vi "自定义成像色谱20200214.vi"(3 "错误输入（无错误）":errorcluster) -> (6 "Color palette":T1(array[cluster]), 7 "生成的色谱条":T2(plugin-control))   [LabVIEW 2018]
uses:
  <vilib>/vision/NI_Vision_Development_Module.lvlib
panel:
  out "对应幅值":dbl[](array[numeric])=[0.0, 0.0, 0.0, 0.0, 255.0, 128.0, 255.0] format="%#.1f%%"
  in  "确 定":bool
  in  "色阶":u32=6 min=2 max=32
  in  "自定义颜色梯度":u32[](array[colorbox])=[8388608, 16744448, 14276864, 32768, 8454143, 16512, 16777215]
  # "自定义显示颜色"
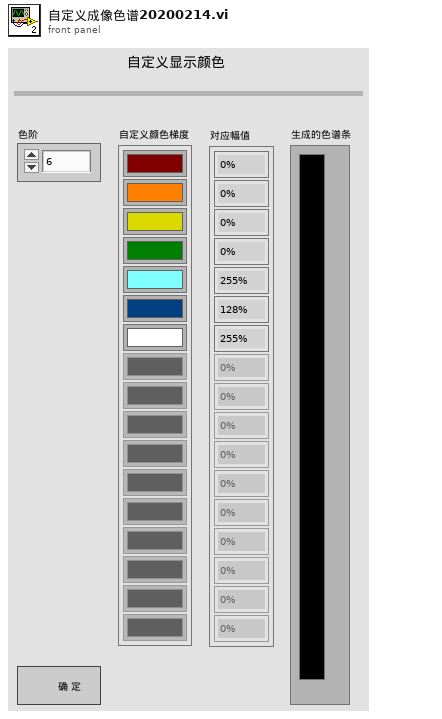
[diagram p1: front panel]
types:
  T1 = cluster{"Red (or Hue) value":u8, "Green (or Sat) value":u8, "Blue (or Light or Val) value":u8}[]
  T2 = typedef "IMAQ Image.ctl" = refnum<image>
  T3 = typedef "Image Type" = u32
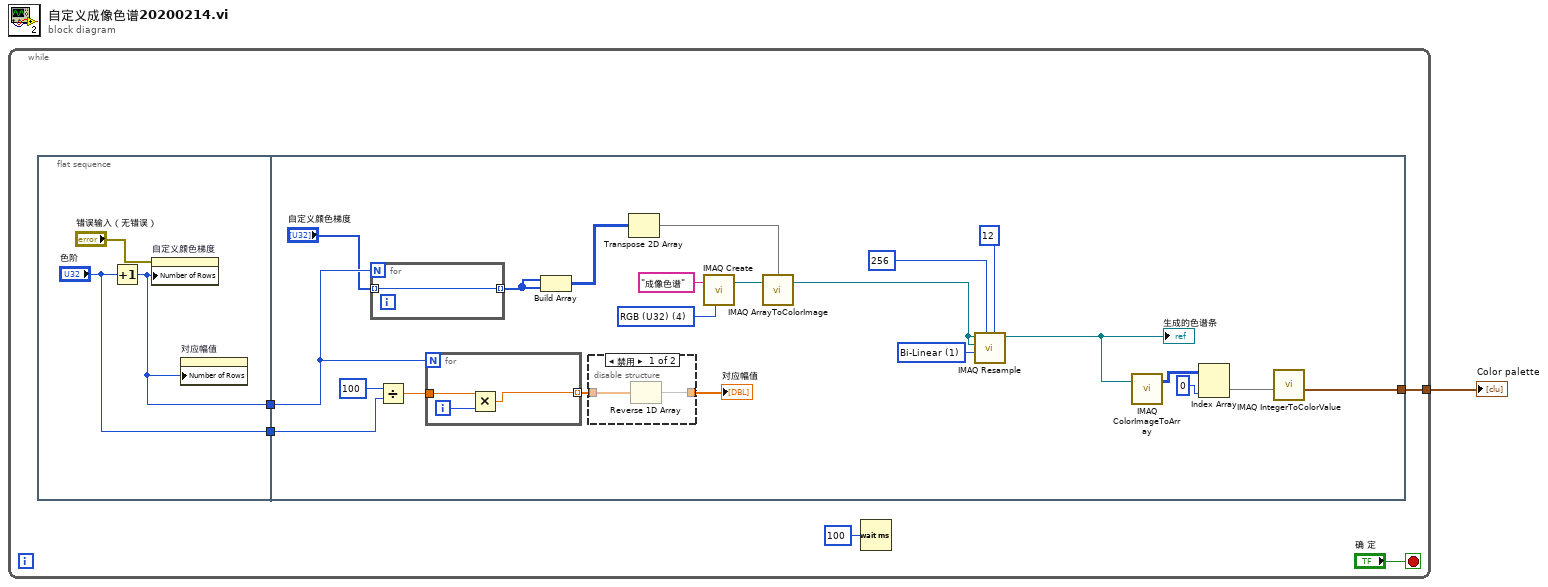
[diagram p0: block diagram]
diagram:
  n1 = while {
    tunnel: [w5] -> w1
    stop <- "确 定" stop-if-true
    n2 = flat-sequence {
      tunnel: [w9] -> w3
      tunnel: ["色阶"] -> w2
      tunnel: [w18] -> w5
      tunnel: w3 -> [w13]
      tunnel: w2 -> [w10]
      frame #0 {
        n3 = Increment(x="色阶") -> (x+1=w9:u32)
        n4 = property on="自定义颜色梯度" class="Arr (严格)"(error in="错误输入（无错误）", "Number of Rows"=w9) -> ()  [unwired: 1 in, 2 out]
        n5 = property on="对应幅值" class="Arr (严格)"("Number of Rows"=w9) -> ()  [unwired: 2 in, 2 out]
      }
      frame #1 {
        w29 = u32 1 items=["Zero Order", "Bi-Linear", "Quadratic", "Cubic Spline"] ("Interpolation Type")
        w30 = T3 4 items=["Grayscale (U8)", "Grayscale (I16)", "Grayscale (SGL)", "Complex (CSG)", "RGB (U32)", "HSL (U32)", "RGB (U64)", "Grayscale (U16)"] ("Image Type")
        n6 = for {
          N: w13 -> [_]
          tunnel: "自定义颜色梯度" -> [w35] mode=indexing
          tunnel: [w35] -> w11 mode=indexing
        }
        n7 = Divide(x=100, y=w10) -> (x/y=w17:dbl)
        n8 = for {
          N: w13 -> [_]
          tunnel: w17 -> [w37]
          tunnel: [w36] -> w15 mode=indexing
          i -> [w38]
          n9 = Multiply(x=w37, y=w38) -> (x*y=w36:dbl)
        }
        n10 = Build Array(w11, w11) -> (w26:u32[][])
        n11 = disable-structure shown="禁用" {
          disable-tunnel: w15 -> [w33 w34]
          disable-tunnel: [w32 w34] -> w14
          frame Disabled {
            n12 = Reverse 1D Array(array=w33) -> (reversed array=w32:dbl[])
          }
          frame Enabled {
          }
        }
        "对应幅值" <- w14
        n13 = Transpose 2D Array(2D array=w26) -> (transposed array=w25:u32[][])
        n14 = call "IMAQ Create"("Image Name"="成像色谱", "Image Type"=w30) -> ("New Image"=w23:T2)  [unwired: 3 in, 1 out]
        n15 = call "IMAQ ArrayToColorImage"("Image Pixels (U32)"=w25, "Image"=w23) -> ("Image Out"=w24:T2)  [unwired: 3 in, 1 out]
        n16 = call "IMAQ Resample"("X Resolution"=12 ("Y Resolution"), "Y Resolution"=256, "Interpolation Type"=w29, "Image Dst"=w24, "Image Src"=w24) -> ("Image Dst Out"=w22:T2)  [unwired: 5 in, 1 out]
        "生成的色谱条" <- w22
        n17 = call "IMAQ ColorImageToArray"("Image"=w22) -> ("Image Pixels (U32)"=w21:u32[][])  [unwired: 3 in, 2 out]
        n18 = Index Array(array=w21, index (col)=0 ("索引 (行)")) -> (element=w19:u32[])  [unwired: 1 in]
        n19 = call "IMAQ IntegerToColorValue"("1D U32 array"=w19) -> ("1D Color value array"=w18:T1)  [unwired: 4 in, 3 out]
      }
    }
    n20 = Wait (ms)(milliseconds to wait=u32 100 ("等待时间（毫秒）")) -> ()  [unwired: 1 out]
  }
  "Color palette" <- w1
